vi "VisualizeAppRingdown.vi"() -> ()   [LabVIEW 2017, in "Visualization.lvlib" / "VisualizeAppRingdown.lvclass"]
uses:
  VisualizeAppRingdown.lvclass
  Modules/AppPlugins/RingdownPlugin/PublicAPI/TypeDef/RingdownOutput.ctl
  C:/dev/Work/PARTF/Visualization/VisualizeApp_class/VisualizeAppBase_class.lvclass
  Modules/AppModule/PublicAPI/Arguments/Broadcasts/clStatUpdate.ctl
  VisializeBase_class/Requests/clUserEventType.ctl
  Modules/EventPlugins/EventPluginBaseClass/TypeDefs/clEvtReportArray.ctl
  Modules/EventPlugins/EventPluginBaseClass/TypeDefs/clEvtReport.ctl
  VisualizeAppBase_class.lvclass/VisualizeAppBase_class.ctl
  VisualizeAppRingdown.lvclass/VisualizeAppRingdown.ctl
  <vilib>/event_ctls.llb/usereventprio.ctl
  VisualizeAppBase/Accessors/Write clEvtReportArray.vi
  Accessors/Write EvtParams.vi
  Accessors/Read EvtParams.vi
  VisualizeAppBase/Accessors/Read clEvtReportArray.vi
  Accessors/Write AppOutput.vi
  Accessors/Read AppOutput.vi
  <vilib>/Utility/error.llb/Error Cluster From Error Code.vi
  <vilib>/express/express shared/transition.llb/Dynamic To Waveform Array.vi
  <vilib>/express/express signal manip/GetorSetDDTAttributes/Set DDT Attributes/SetT0.vi
  <vilib>/express/express shared/transition.llb/Waveform Array To Dynamic.vi
  <vilib>/ErrorRing/Error Ring.xnode
  <vilib>/express/express signal manip/GetorSetDDTAttributes/Set DDT Attributes/Set DDT Properties.xnode
  <userlib>/NIST/NISTErrorLib/NISTErrorLib.lvlib
  VisializeBase_class/VisualizeBase_class.lvclass
  Modules/AppModule/AppModule.lvlib
  Modules/EventPlugins/EventPluginBaseClass/EventPluginBaseClass.lvclass
  Modules/AppPlugins/RingdownPlugin/RingdownPlugin.lvclass
  Modules/PmuImpairModule/PmuImpairModule.lvlib
  Modules/EventModule/EventModule.lvlib
panel:
  out "ActivePlot":u32=1
  out "Timeoffset":dbl=1e+32
  in  "restart VI":bool
  out "Error Array":errorcluster[][](array[cluster])
  out "Active Power Signal":dynamicdata(graph)
  out "Error signal":waveform(dbl)[](graph)
  out "S Plane":cluster{"Damping":dbl[], "Frequency":dbl[]}[](graph)
  in  "Number of Visible Modes":dbl=5.0
  out "Input Data":dbl[][](array[numeric])
  out "data 2":T1
  in  "QueName":string="VisAppQue"
  in  "btnStop":bool
  out "Status Broadcasts":string
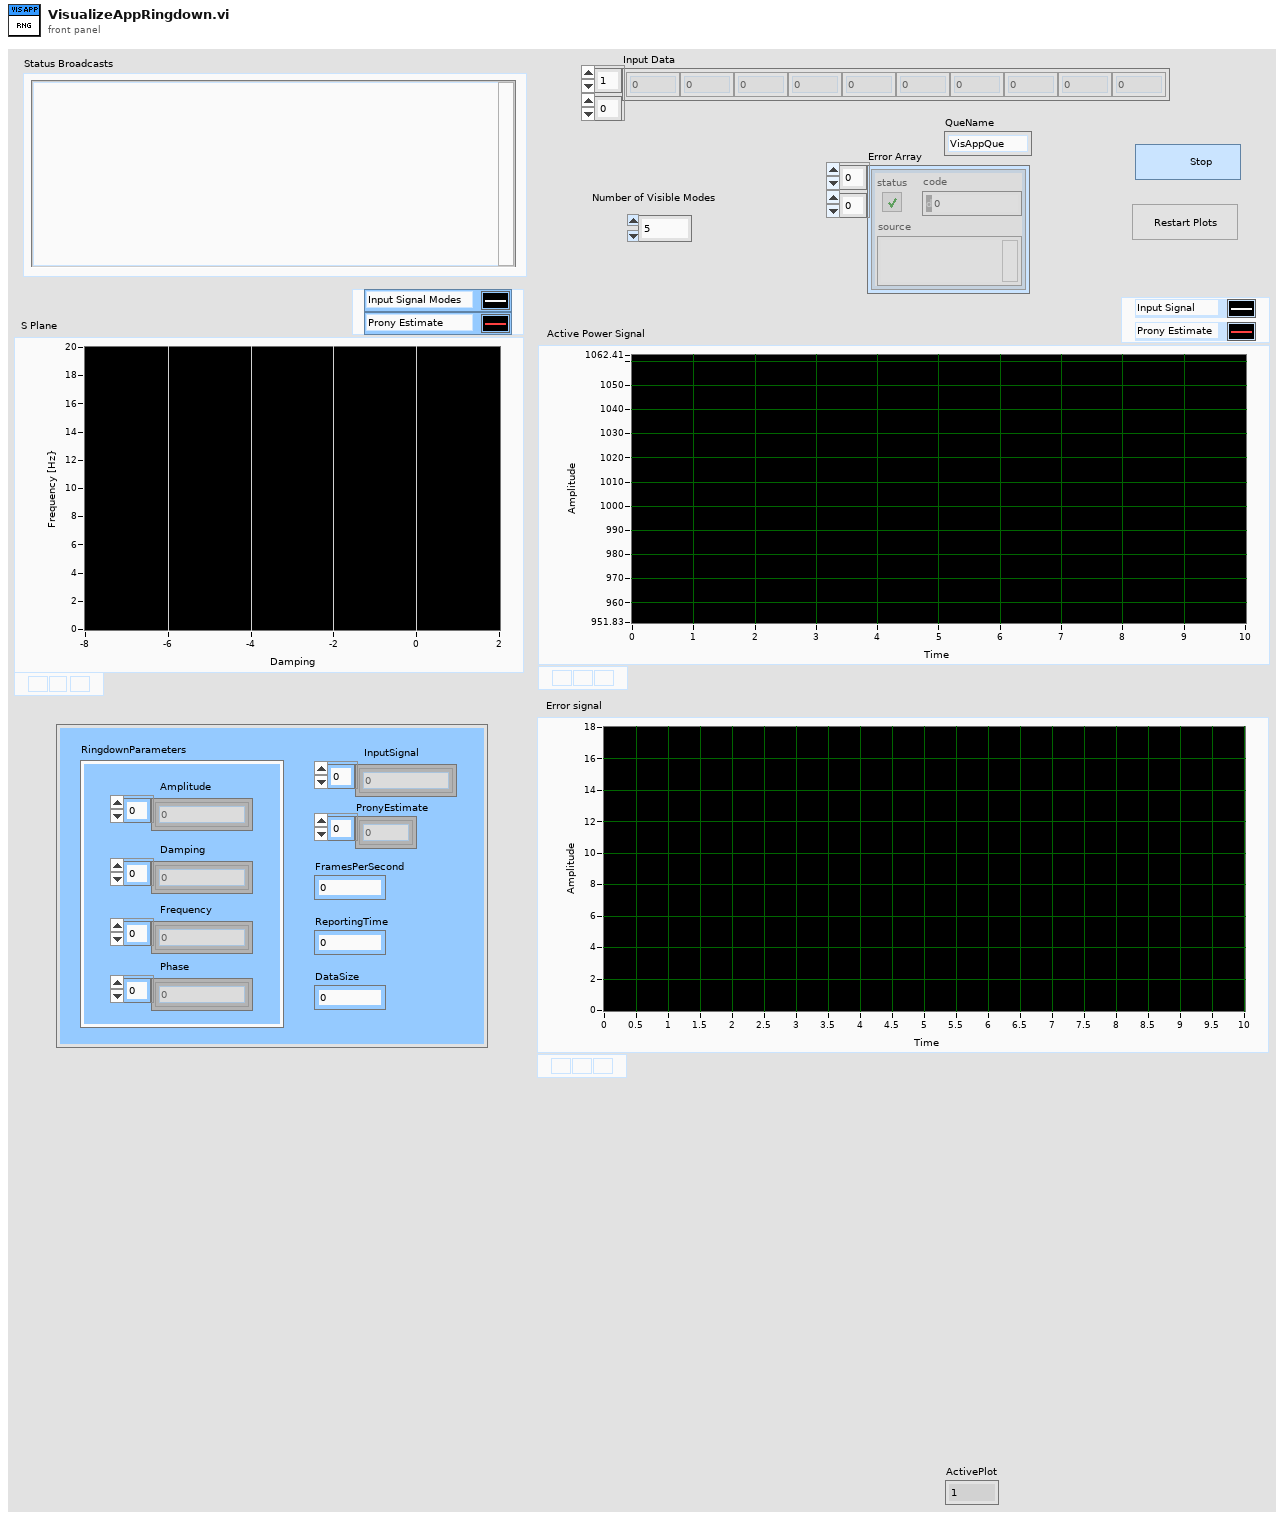
[diagram p1: front panel]
types:
  T1 = typedef "AppPlugins.lvlib/RingdownPlugin.lvclass/RingdownOutput.ctl" = cluster{"FramesPerSecond":dbl, "PronyEstimate":dbl[], "RingdownParameters":cluster{"Amplitude":dbl[], "Damping":dbl[], "Frequency":dbl[], "Phase":dbl[]}, "ReportingTime":dbl, "DataSize":u32, "InputSignal":dbl[]}
  T2 = typedef "EventPlugins.lvlib/EventPluginBaseClass.lvclass/clEvtReportArray.ctl" = T3[]
  T3 = typedef "EventPlugins.lvlib/EventPluginBaseClass.lvclass/clEvtReport.ctl" = cluster{"Timestamp":dbl, "Synx":cdb[], "Freq":dbl, "ROCOF":dbl, "ID":i16}
  T4 = typedef "Visualization.lvlib/VisualizeBase_class.lvclass/clUserEventType.ctl" = cluster{"BusIndex":i8, "Data":variant}
  T5 = typedef "usereventprio.ctl" = enum32{"high priority", "normal priority"}
  T6 = typedef "AppModule.lvlib/clStatUpdate.ctl" = cluster{"Status":string}
  T7 = typedef "Visualization.lvlib/VisualizeBase_class.lvclass/clRequestEvents.ctl" = cluster{"StopRequest":refnum<user-event>}
  T8 = typedef "AppModule.lvlib/clBroadcastEvents.ctl" = cluster{"DidInit":refnum<user-event>, "StatusUpdate":refnum<user-event>, "ErrorReport":refnum<user-event>, "DidStop":refnum<user-event>, "PathToINI":refnum<user-event>, "InputData":refnum<user-event>, "OutputData":refnum<user-event>, "BcAppInfo":refnum<user-event>, "ConfigData":refnum<user-event>}
  T9 = typedef "PmuImpairModule.lvlib/clBroadcastEvents.ctl" = cluster{"DidInit":refnum<user-event>, "StatusUpdate":refnum<user-event>, "ErrorReport":refnum<user-event>, "DidStop":refnum<user-event>, "ImpairConfig":refnum<user-event>, "ImpairParams":refnum<user-event>, "ImpairReports":refnum<user-event>, "PathToPlugin":refnum<user-event>, "BusNumber":refnum<user-event>}
  T10 = typedef "EventModule.lvlib/clBroadcastEvents.ctl" = cluster{"DidInit":refnum<user-event>, "StatusUpdate":refnum<user-event>, "ErrorReport":refnum<user-event>, "DidStop":refnum<user-event>, "ReadEvtConfig":refnum<user-event>, "ReadTimeArray":refnum<user-event>, "ReadEvtParams":refnum<user-event>, "GetEvtReportArray":refnum<user-event>, "ReadPathToPlugin":refnum<user-event>, "GetEvtSignal":refnum<user-event>, "ReadBusNumber":refnum<user-event>}
  T11 = cluster{"Amplitude":dbl[], "Damping":dbl[], "Frequency":dbl[], "Phase":dbl[]}
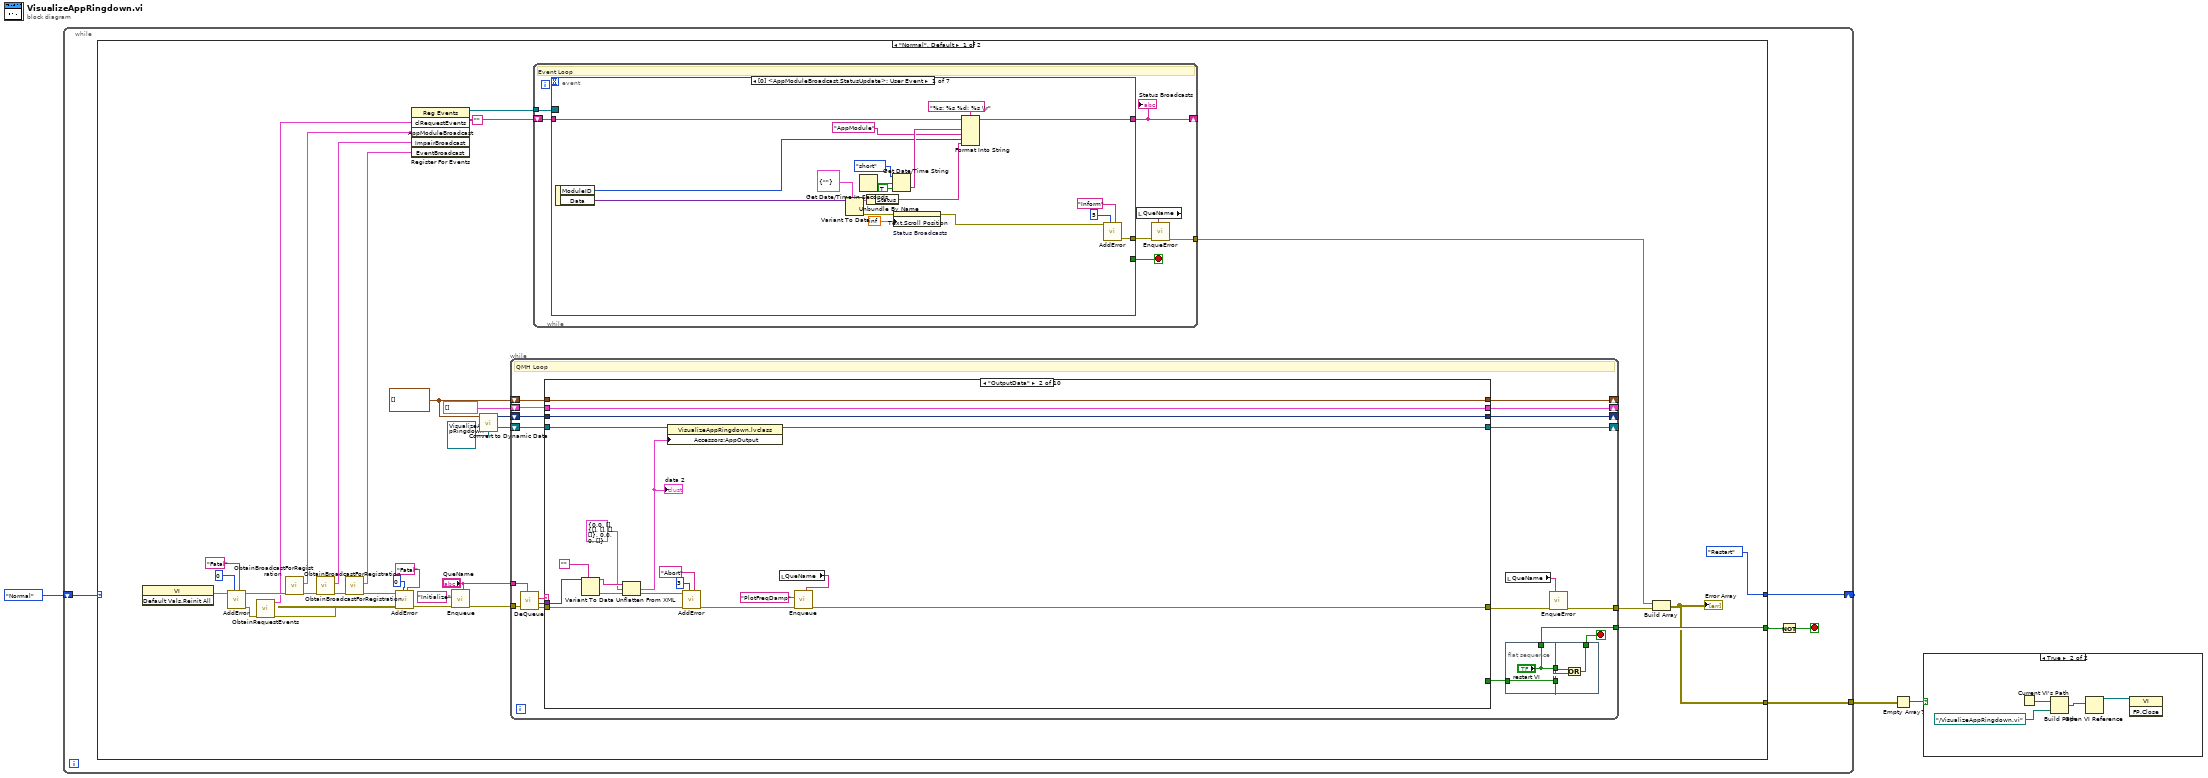
[diagram p0: block diagram]
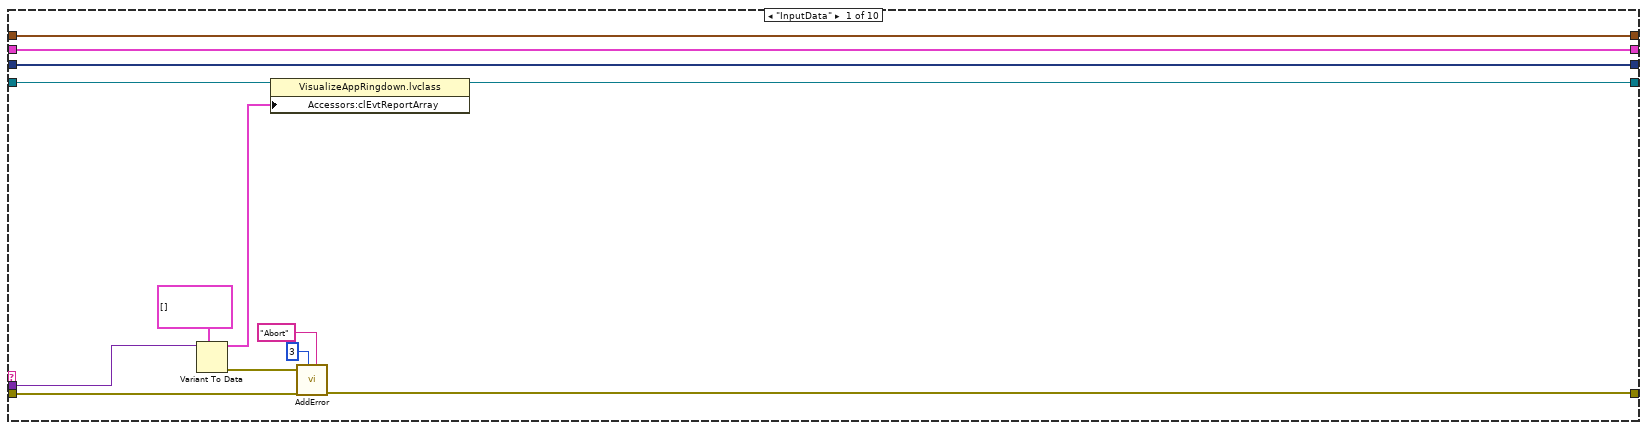
[diagram p3: hidden frame]
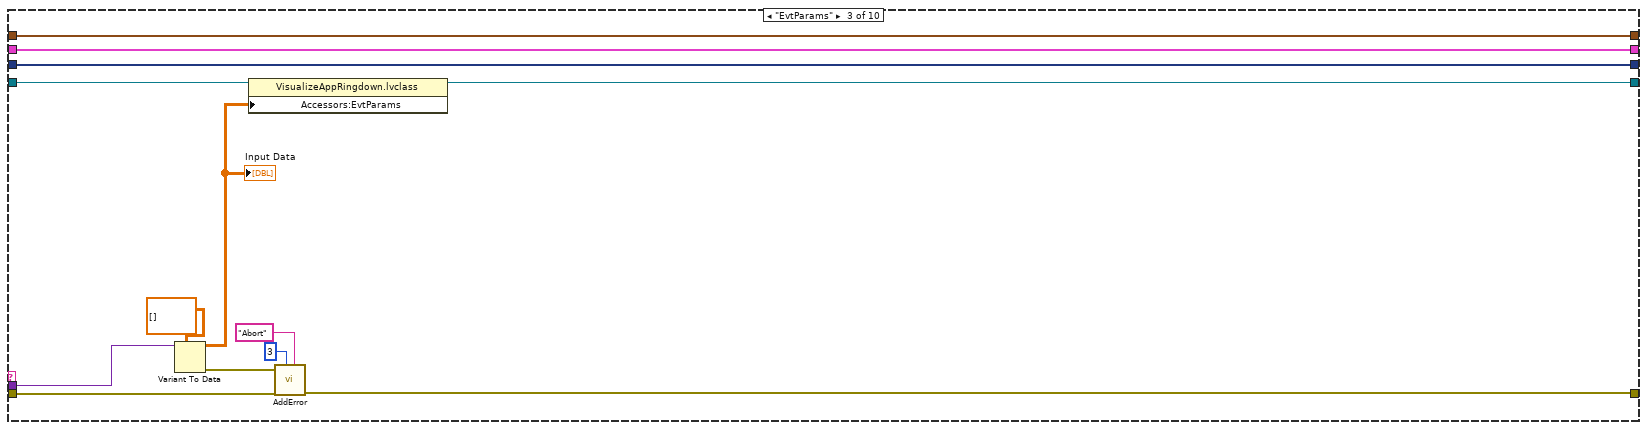
[diagram p4: hidden frame]
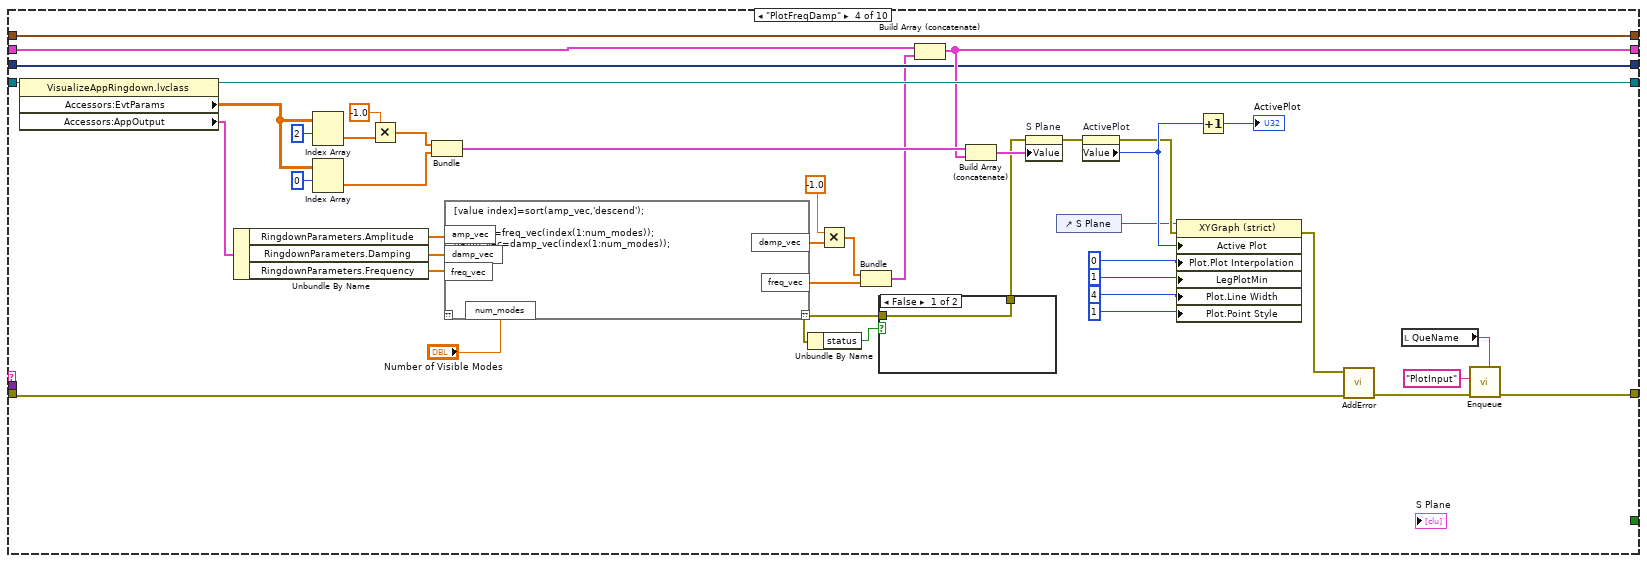
[diagram p5: hidden frame]
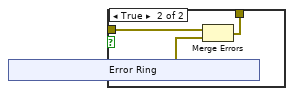
[diagram p6: hidden frame]
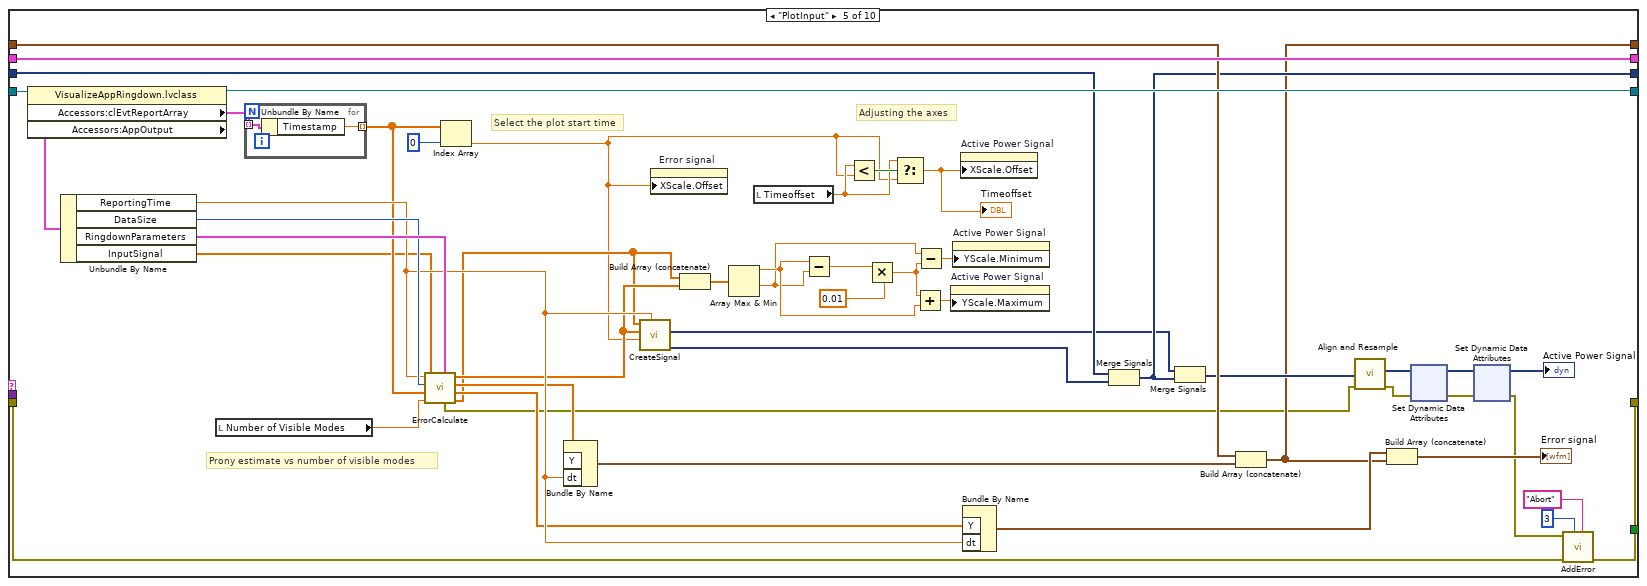
[diagram p7: hidden frame]
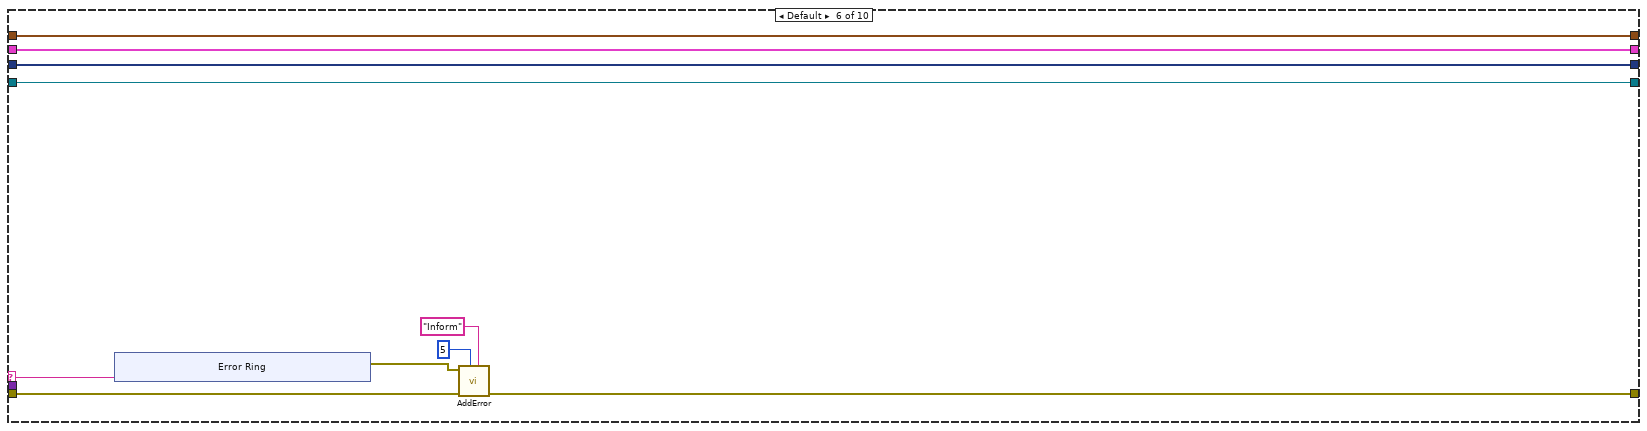
[diagram p8: hidden frame]
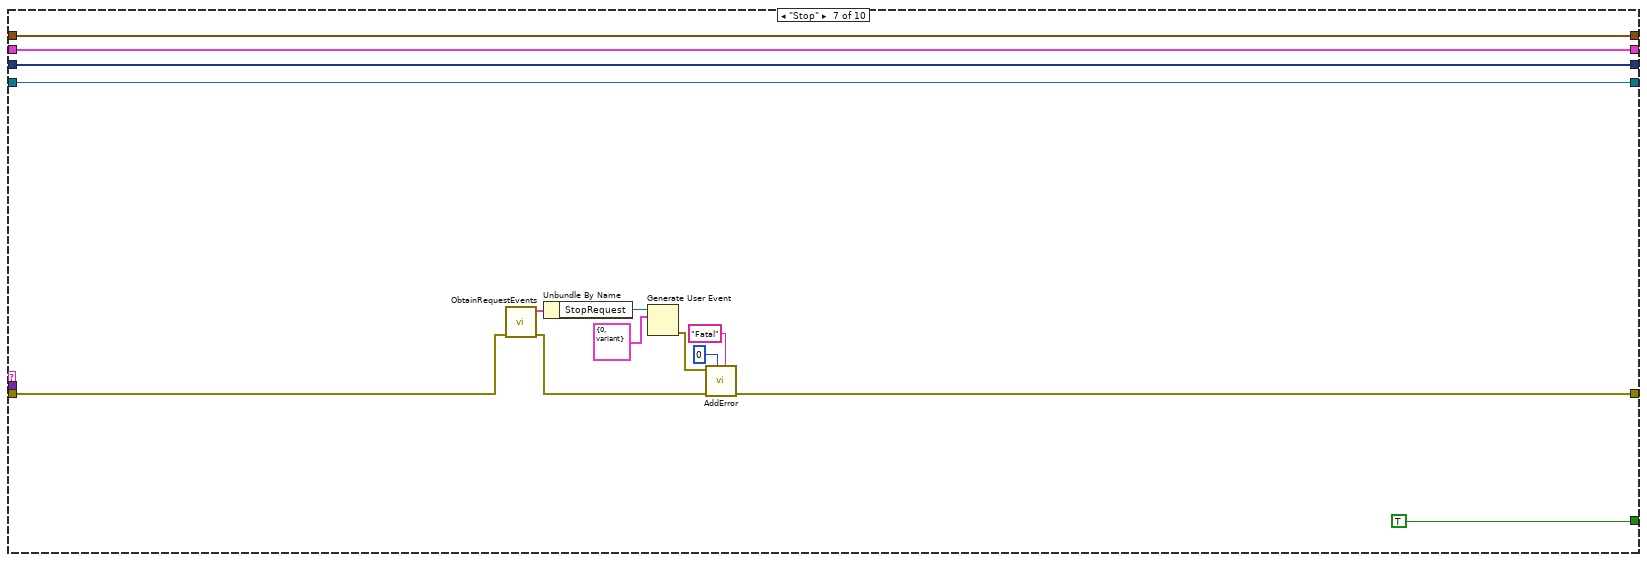
[diagram p9: hidden frame]
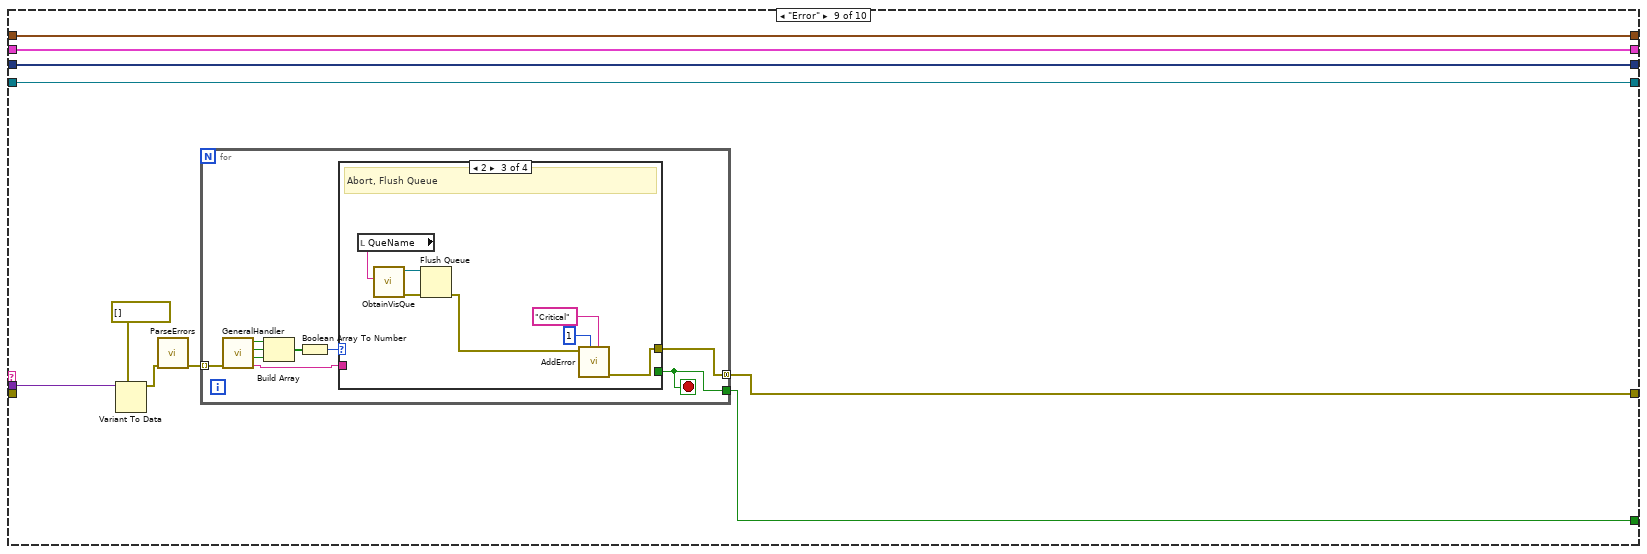
[diagram p11: hidden frame]
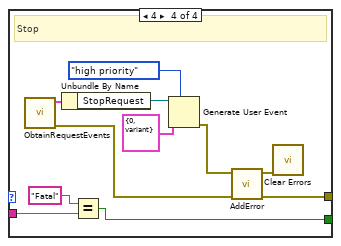
[diagram p14: hidden frame]
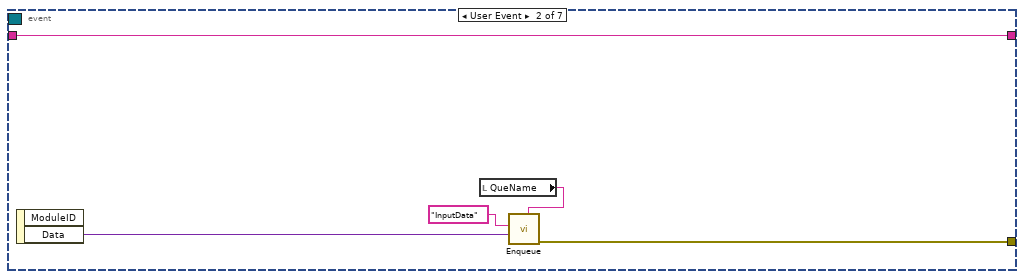
[diagram p16: hidden frame]
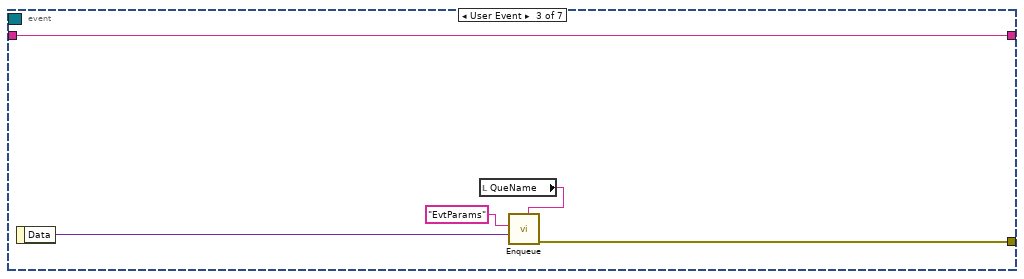
[diagram p17: hidden frame]
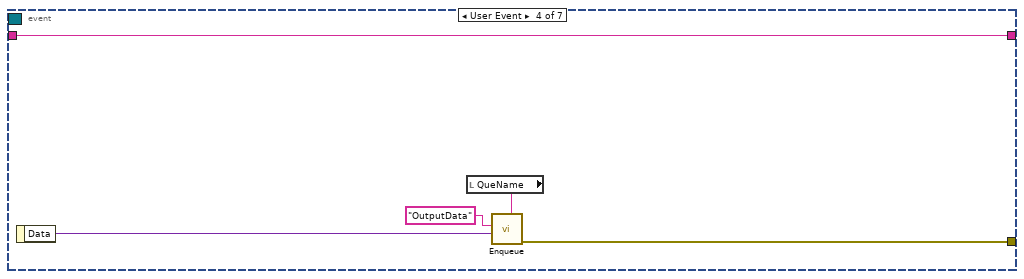
[diagram p18: hidden frame]
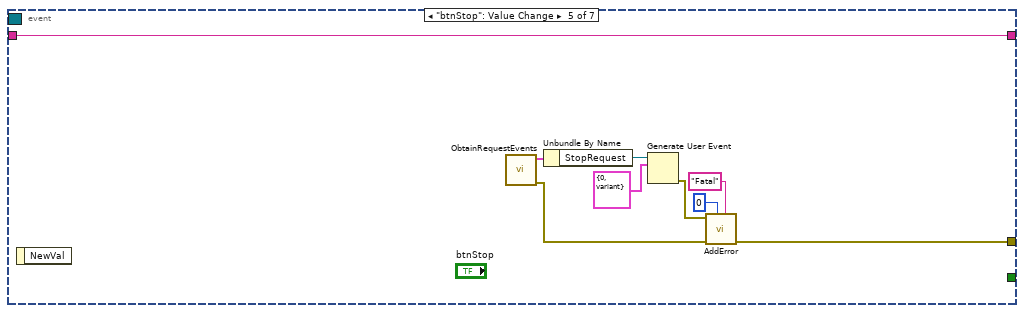
[diagram p19: hidden frame]
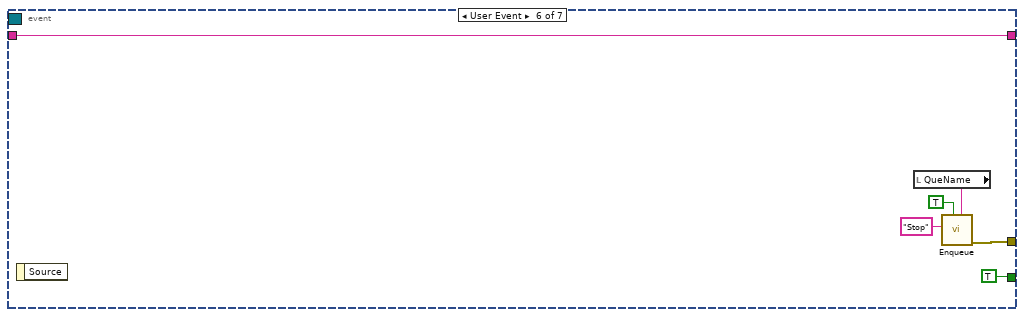
[diagram p20: hidden frame]
diagram:
  n1 = while {
    shift-right: [w5] -> _
    shift-left: enum16{"Normal", "Restart"}."Normal" -> [w6]
    tunnel: [w4] -> w1
    stop <- w7 stop-if-true
    n2 = case shown="\"Normal\", Default" w6 {
      tunnel: [w13 TRUE] -> w8
      tunnel: [enum16{"Normal", "Restart"}."Restart" enum16{"Normal", "Restart"}."Normal"] -> w5
      tunnel: [w9 errorcluster[][] []] -> w4
      frame "Normal", Default {
        w11 = waveform(dbl)[] []
        n3 = invoke class="VI" method="Default Vals.Reinit All"() -> (error out=w21:errorcluster)  [unwired: 3 in, 2 out]
        n4 = call <userlib>:"AddError.vi"("Severity"="Fatal", "Priority"=u8 0, "error in (no error)"=w21) -> ("ErrorArray"=w36:errorcluster[], "error out"=w35:errorcluster)  [unwired: 7 in]
        n5 = call "ObtainRequestEvents.vi"("Error"=w36) -> ("Error"=w32:errorcluster[], "clRequestEvents"=w34:T7)  [unwired: 9 in]
        n6 = call "ObtainBroadcastForRegistration.vi"("error in (no error)"=w35) -> ("error out"=w20:errorcluster, "AppModuleBroadcast"=w33:T8)  [unwired: 9 in]
        n7 = call "ObtainBroadcastForRegistration.vi"("error in (no error)"=w20) -> ("error out"=w19:errorcluster, "ImpairBroadcast"=w18:T9)  [unwired: 9 in]
        n8 = call "ObtainBroadcastForRegistration.vi"("error in (no error)"=w19) -> ("error out"=w16:errorcluster, "EventBroadcast"=w15:T10)  [unwired: 9 in]
        n9 = call <userlib>:"AddError.vi"("Severity"="Fatal", "Priority"=u8 0, "ErrorArray"=w32, "error in (no error)"=w16) -> ("ErrorArray"=w30:errorcluster[])  [unwired: 6 in, 1 out]
        n10 = register-events(w34, w33, w18, w15) -> (reference out=w25:refnum<event-registration>)  [unwired: 2 in, 1 out]
        n11 = call "Enqueue.vi"("QueName"="QueName", "Error"=w30, "Message"="Initialize") -> ("Error"=w27:errorcluster[])  [unwired: 8 in]
        n12 = call "Convert to Dynamic Data"("Array of Waveforms"=w11) -> ("Dynamic Data Type"=w10:dynamicdata)  [unwired: 3 in]
        n13 = while {
          tunnel: w27 -> [w59]
          tunnel: "QueName" -> [w58]
          tunnel: [w52] -> w24
          shift-right: [w50] -> _
          shift-left: refnum<class "VisualizeAppRingdown.lvclass"> refnum ("Visualization.lvlib:VisualizeAppRingdown.lvclass") -> [w51]
          shift-right: [w49] -> _
          shift-left: cluster{"Damping":dbl[], "Frequency":dbl[]}[] [] -> [w48]
          shift-right: [w46] -> _
          shift-left: w10 -> [w47]
          shift-right: [w44] -> _
          shift-left: w11 -> [w45]
          tunnel: [w43] -> w13
          stop <- w39 stop-if-true
          # "QMH Loop"
          n14 = call "DeQueue.vi"("QueName"=w58, "Error"=w59) -> ("Error"=w55:errorcluster[], "Data"=w56:variant, "Message"=w57:string)  [unwired: 7 in]
          n15 = case shown="\"OutputData\"" w57 {
            selector: w57 -> [_ _ _ _ _ w250 _ _ _ _]
            tunnel: w56 -> [w75 w94 w107 _ _ _ _ _ w283 _]
            tunnel: w55 -> [w71 w93 w104 w122 w174 w249 w263 w276 _ w314]
            tunnel: [w70 w89 w103 w119 w173 w245 w264 w276 w285 w314] -> w54
            tunnel: [_ _ _ _ _ _ TRUE _ w286 _] -> w41
            tunnel: w51 -> [w77 w96 w109 w152 w210 w244 w261 w275 w280 w315]
            tunnel: [w76 w95 w108 w151 w209 w244 w261 w275 w280 w315] -> w50
            tunnel: [w67 w86 w99 w143 w208 w243 w260 w274 w279 w317] -> w49
            tunnel: w48 -> [w67 w86 w99 w144 w208 w243 w260 w274 w279 w317]
            tunnel: w47 -> [w66 w85 w98 w142 w201 w242 w259 w273 w278 w316]
            tunnel: [w66 w85 w98 w142 w200 w242 w259 w273 w278 w316] -> w46
            tunnel: w45 -> [w65 w84 w97 w140 w205 w241 w258 w272 w277 w318]
            tunnel: [w65 w84 w97 w140 w198 w241 w258 w272 w277 w318] -> w44
            frame "InputData" {
              n16 = Variant To Data(type=T2 [] ("clEvtReportArray"), Variant=w75) -> (data=w73:T2, error out=w72:errorcluster)  [unwired: 1 in]
              n17 = property class="VisualizeAppRingdown.lvclass"(reference=w77, "Accessors:clEvtReportArray"=w73) -> (reference out=w76:refnum<class "VisualizeAppRingdown.lvclass">)  [unwired: 1 in, 1 out]
              n18 = call <userlib>:"AddError.vi"("Severity"="Abort", "Priority"=u8 3, "ErrorArray"=w71, "error in (no error)"=w72) -> ("ErrorArray"=w70:errorcluster[])  [unwired: 6 in, 1 out]
            }
            frame "OutputData" {
              n19 = Variant To Data(type="", Variant=w94) -> (data=w83:string, error out=w80:errorcluster)  [unwired: 1 in]
              n20 = Unflatten From XML(xml string=w83, type=T1 {"FramesPerSecond"=0.0, "PronyEstimate"=[], "RingdownParameters"={"Amplitude"=[], "Damping"=[], "Frequency"=[], "Phase"=[]}, "ReportingTime"=0.0, "DataSize"=0, "InputSignal"=[]} ("RingdownOutput"), error in (no error)=w80) -> (value=w78:T1, error out=w79:errorcluster)
              "data 2" <- w78
              n21 = property class="VisualizeAppRingdown.lvclass"(reference=w96, "Accessors:AppOutput"=w78) -> (reference out=w95:refnum<class "VisualizeAppRingdown.lvclass">)  [unwired: 1 in, 1 out]
              n22 = call <userlib>:"AddError.vi"("Severity"="Abort", "Priority"=u8 3, "ErrorArray"=w93, "error in (no error)"=w79) -> ("ErrorArray"=w90:errorcluster[])  [unwired: 6 in, 1 out]
              n23 = local read "QueName"() -> (w87:string)
              n24 = call "Enqueue.vi"("QueName"=w87, "Error"=w90, "Message"="PlotFreqDamp") -> ("Error"=w89:errorcluster[])  [unwired: 8 in]
            }
            frame "EvtParams" {
              n25 = Variant To Data(type=dbl[][] [], Variant=w107) -> (data=w106:dbl[][], error out=w105:errorcluster)  [unwired: 1 in]
              "Input Data" <- w106
              n26 = property class="VisualizeAppRingdown.lvclass"(reference=w109, "Accessors:EvtParams"=w106) -> (reference out=w108:refnum<class "VisualizeAppRingdown.lvclass">)  [unwired: 1 in, 1 out]
              n27 = call <userlib>:"AddError.vi"("Severity"="Abort", "Priority"=u8 3, "ErrorArray"=w104, "error in (no error)"=w105) -> ("ErrorArray"=w103:errorcluster[])  [unwired: 6 in, 1 out]
            }
            frame "PlotFreqDamp" {
              n28 = property class="VisualizeAppRingdown.lvclass"(reference=w152) -> (reference out=w151:refnum<class "VisualizeAppRingdown.lvclass">, "Accessors:EvtParams"=w148:dbl[][], "Accessors:AppOutput"=w150:T1)  [unwired: 1 in, 1 out]
              n29 = Unbundle By Name(w150) -> ("RingdownParameters.Amplitude"=w132:dbl[], "RingdownParameters.Damping"=w131:dbl[], "RingdownParameters.Frequency"=w130:dbl[])
              n30 = Index Array(array=w148, index (row)=2) -> (element=w139:dbl[])  [unwired: 1 in]
              n31 = Index Array(array=w148, index (row)=0) -> (element=w146:dbl[])  [unwired: 1 in]
              n32 = Multiply(x=-1.0, y=w139) -> (x*y=w138:dbl[])
              n33 = Bundle(w138, "Accessors:EvtParams"=w146) -> (w145:cluster{dbl[], "Accessors:EvtParams":dbl[]})  [unwired: 1 in]
              n34 = script code="[value index]=sort(amp_vec,'descend');\n\nfreq_vec=freq_vec(index(1:num_modes));\ndamp_vec=damp_vec(index(1:num_modes));"("amp_vec"=w132, "damp_vec"=w131, "freq_vec"=w130, "num_modes"="Number of Visible Modes") -> ("??"=w111:errorcluster, "damp_vec"=w134:dbl[], "freq_vec"=w133:dbl[])  [unwired: 1 in]
              n35 = Unbundle By Name(w111) -> ("status"=w110:bool)
              n36 = Multiply(x=-1.0, y=w134) -> (x*y=w135:dbl[])
              n37 = Bundle(w135, w133) -> (w141:cluster{dbl[], dbl[]})  [unwired: 1 in]
              n38 = case shown="False" w110 {
                tunnel: [w153 w156] -> w112
                tunnel: w111 -> [w153 w154]
                frame False {
                }
                frame True {
                  n39 = xnode "Error Ring"() -> ("error out"=w155:errorcluster)
                  n40 = Merge Errors(w154, w155) -> (w156:errorcluster)
                }
              }
              n41 = Build Array (concatenate)(w144, w141) -> (w143:cluster{"Damping":dbl[], "Frequency":dbl[]}[])
              n42 = Build Array (concatenate)(w145, w143) -> (w127:cluster{"Damping":dbl[], "Frequency":dbl[]}[])
              n43 = property on="S Plane" class="XYGraph (strict)"(error in=w112, "Value"=w127) -> (error out=w126:errorcluster)  [unwired: 1 in, 1 out]
              n44 = control-ref of="S Plane"() -> (w113:refnum<vi>)
              n45 = property on="ActivePlot" class="DigNum (strict)"(error in=w126) -> (error out=w124:errorcluster, "Value"=w125:u32)  [unwired: 1 in, 1 out]
              n46 = property on="Property Node" class="XYGraph (strict)"(reference=w113, error in=w124, "Active Plot"=w125, "Plot.Plot Interpolation"=u8 0, "LegPlotMin"=u32 1 ("Legend:Plot Minimum"), "Plot.Line Width"=u8 4, "Plot.Point Style"=u8 1) -> (error out=w123:errorcluster)  [unwired: 1 out]
              n47 = Increment(x=w125) -> (x+1=→"ActivePlot":u32)
              n48 = call <userlib>:"AddError.vi"("ErrorArray"=w122, "error in (no error)"=w123) -> ("ErrorArray"=w120:errorcluster[])  [unwired: 8 in, 1 out]
              n49 = local read "QueName"() -> (w118:string)
              n50 = call "Enqueue.vi"("QueName"=w118, "Error"=w120, "Message"="PlotInput") -> ("Error"=w119:errorcluster[])  [unwired: 8 in]
            }
            frame "PlotInput" {
              # "Adjusting the axes"
              # "Select the plot start time"
              # "Prony estimate vs number of visible modes"
              n51 = property class="VisualizeAppRingdown.lvclass"(reference=w210) -> (reference out=w209:refnum<class "VisualizeAppRingdown.lvclass">, "Accessors:clEvtReportArray"=w193:T2, "Accessors:AppOutput"=w207:T1)  [unwired: 1 in, 1 out]
              n52 = Unbundle By Name(w207) -> ("ReportingTime"=w178:dbl, "DataSize"=w179:u32, "RingdownParameters"=w180:T11, "InputSignal"=w164:dbl[])
              n53 = local read "Number of Visible Modes"() -> (w166:dbl)
              n54 = for {
                tunnel: w193 -> [w240] mode=indexing
                tunnel: [w239] -> w167 mode=indexing
                n55 = Unbundle By Name(w240) -> ("Timestamp"=w239:dbl)
              }
              n56 = call "ErrorCalculate.vi"("RingdownParameters"=w180, "input_data"=w164, "num_modes"=w166, "time"=w167, "nnfit"=w179, "dft"=w178) -> ("input_data"=w163:dbl[], "null_input"=w177:dbl[], "error_sig"=w175:dbl[], "prony_estimate"=w176:dbl[], "error out"=w165:errorcluster)  [unwired: 1 in]
              n57 = Index Array(array=w167, index=0) -> (element=w162:dbl)
              n58 = Bundle By Name("Y"=w175, "dt"=w178) -> (w206:waveform(dbl))  [unwired: 1 in]
              n59 = call "CreateSignal.vi"("dt"=w178, "t0_1"=w162, "PronyEstimate"=w176, "InputSignal"=w163) -> ("DynamicPronyEstimate"=w181:dynamicdata, "DynamicInputSignal"=w182:dynamicdata)  [unwired: 6 in]
              n60 = property on="Error signal" class="WFGraph (strict)"("XScale.Offset"=w162) -> ()  [unwired: 2 in, 2 out]
              n61 = Build Array (concatenate)(w163, w176) -> (w186:dbl[])
              n62 = Array Max & Min(array=w186) -> (max value=w190:dbl, min value=w189:dbl)  [unwired: 2 out]
              n63 = local read "Timeoffset"() -> (w196:dbl)
              n64 = Subtract(x=w190, y=w189) -> (x-y=w188:dbl)
              n65 = Less?(x=w196, y=w162) -> (x < y?=w197:bool)
              n66 = Multiply(x=w188, y=0.01) -> (x*y=w187:dbl)
              n67 = Select(t=w196, s=w197, f=w162) -> (s? t:f=w194:dbl)
              "Timeoffset" <- w194
              n68 = Add(x=w187, y=w190) -> (x+y=w192:dbl)
              n69 = Subtract(x=w189, y=w187) -> (x-y=w195:dbl)
              n70 = property on="Active Power Signal" class="WFGraph (strict)"("YScale.Maximum"=w192) -> ()  [unwired: 2 in, 2 out]
              n71 = property on="Active Power Signal" class="WFGraph (strict)"("YScale.Minimum"=w195) -> ()  [unwired: 2 in, 2 out]
              n72 = property on="Active Power Signal" class="WFGraph (strict)"("XScale.Offset"=w194) -> ()  [unwired: 2 in, 2 out]
              n73 = Bundle By Name("Y"=w177, "dt"=w178) -> (w203:waveform(dbl))  [unwired: 1 in]
              n74 = Merge Signals(w201, w181) -> (w200:dynamicdata)
              n75 = Merge Signals(w182, w200) -> (w199:dynamicdata)
              n76 = Build Array (concatenate)(w205, w206) -> (w198:waveform(dbl)[])
              n77 = call "Align and Resample"("error in (no error)"=w165, "Signals"=w199) -> ("error out"=w172:errorcluster, "Resampled Signals"=w185:dynamicdata)  [unwired: 7 in, 1 out]
              n78 = Build Array (concatenate)(w203, w198) -> (→"Error signal":waveform(dbl)[])
              n79 = xnode "Set Dynamic Data Attributes"("Signals In"=w185, "error in"=w172) -> ("Signals Out"=w184:dynamicdata, "error out"=w171:errorcluster)  [unwired: 2 in]
              n80 = xnode ("Set Dynamic Data Attributes")("Signals In"=w184, "error in"=w171) -> ("Signals Out"=→"Active Power Signal":dynamicdata, "error out"=w170:errorcluster)  [unwired: 2 in]
              n81 = call <userlib>:"AddError.vi"("Severity"="Abort", "Priority"=u8 3, "ErrorArray"=w174, "error in (no error)"=w170) -> ("ErrorArray"=w173:errorcluster[])  [unwired: 6 in, 1 out]
            }
            frame Default {
              n82 = xnode "Error Ring"("parameter 0"=w250) -> ("error out"=w248:errorcluster)
              n83 = call <userlib>:"AddError.vi"("Severity"="Inform", "Priority"=u8 5, "ErrorArray"=w249, "error in (no error)"=w248) -> ("ErrorArray"=w245:errorcluster[])  [unwired: 6 in, 1 out]
            }
            frame "Stop" {
              n84 = call "ObtainRequestEvents.vi"("Error"=w263) -> ("Error"=w262:errorcluster[], "clRequestEvents"=w265:T7)  [unwired: 9 in]
              n85 = Unbundle By Name(w265) -> ("StopRequest"=w266:refnum<user-event>)
              n86 = Generate User Event(user event=w266, event data cluster=T4 {"BusIndex"=0, "Data"=variant} ("clEventType")) -> (error out=w268:errorcluster)  [unwired: 2 in, 1 out]
              n87 = call <userlib>:"AddError.vi"("Severity"="Fatal", "Priority"=u8 0, "ErrorArray"=w262, "error in (no error)"=w268) -> ("ErrorArray"=w264:errorcluster[])  [unwired: 6 in, 1 out]
            }
            frame "Initialize" {
            }
            frame "Error" {
              n88 = Variant To Data(type=errorcluster[] [], Variant=w283) -> (data=w281:errorcluster[])  [unwired: 1 in, 1 out]
              n89 = call <userlib>:"ParseErrors.vi"("ErrorArray"=w281) -> ("ErrorArray"=w284:errorcluster[])  [unwired: 8 in, 2 out]
              n90 = for {
                tunnel: w284 -> [w295] mode=indexing
                tunnel: [w289] -> w285 mode=concatenating
                tunnel: [w287] -> w286
                stop <- w287 stop-if-true
                n91 = call <userlib>:"GeneralHandler.vi"("error in (no error)"=w295) -> ("Severity"=w288:string, "Stop"=w292:bool, "Abort"=w293:bool, "Continue"=w294:bool)  [unwired: 7 in]
                n92 = Build Array(w294, w293, w292) -> (w291:bool[])
                n93 = Boolean Array To Number(Boolean array=w291) -> (number=w290:u32)
                n94 = case shown="2" w290 {
                  tunnel: [_ _ w300 w311] -> w289
                  tunnel: w288 -> [_ _ _ w305]
                  tunnel: [_ _ _ w303] -> w287
                  frame 0, Default {
                    # "No Dialog"
                  }
                  frame 1 {
                    # "Continue"
                  }
                  frame 2 {
                    # "Abort, Flush Queue"
                    n95 = local read "QueName"() -> (w296:string)
                    n96 = call "ObtainVisQue.vi"("QueName"=w296) -> ("error out"=w302:errorcluster, "queue out"=w301:refnum<queue>)  [unwired: 9 in]
                    n97 = Flush Queue(queue=w301, error in (no error)=w302) -> (error out=w299:errorcluster)  [unwired: 2 out]
                    n98 = call <userlib>:"AddError.vi"("Severity"="Critical" ("String"), "Priority"=u8 1, "error in (no error)"=w299) -> ("ErrorArray"=w300:errorcluster[])  [unwired: 7 in, 1 out]
                  }
                  frame 4 {
                    # "Stop"
                    n99 = call "ObtainRequestEvents.vi"() -> ("Error"=w309:errorcluster[], "clRequestEvents"=w313:T7)  [unwired: 10 in]
                    n100 = Unbundle By Name(w313) -> ("StopRequest"=w312:refnum<user-event>)
                    n101 = Equal?(x="Fatal", y=w305) -> (x = y?=w303:bool)
                    n102 = Generate User Event(priority (normal)=usereventprio."high priority", user event=w312, event data cluster=T4 {"BusIndex"=0, "Data"=variant} ("event data")) -> (error out=w310:errorcluster)  [unwired: 1 in, 1 out]
                    n103 = call <userlib>:"AddError.vi"("ErrorArray"=w309, "error in (no error)"=w310) -> ("ErrorArray"=w311:errorcluster[], "error out"=w306:errorcluster)  [unwired: 8 in]
                    n104 = call <vilib>:"Clear Errors.vi"("error in (no error)"=w306) -> ()  [unwired: 5 in, 2 out]
                  }
                }
              }
            }
            frame "Restart" {
            }
          }
          n105 = flat-sequence {
            tunnel: ["restart VI"] -> w43
            tunnel: ["restart VI"] -> w42
            tunnel: w41 -> [w60]
            tunnel: [w60] -> w40
            tunnel: w42 -> [w64]
            tunnel: w40 -> [w63]
            tunnel: [w62] -> w39
            frame #0 {
            }
            frame #1 {
              n106 = Or(x=w63, y=w64) -> (x .or. y?=w62:bool)
            }
          }
          n107 = local read "QueName"() -> (w53:string)
          n108 = call "EnqueError.vi"("QueName"=w53, "Error"=w54) -> ("Error"=w52:errorcluster[])  [unwired: 9 in]
        }
        n109 = while {
          tunnel: [w324] -> w23
          tunnel: w25 -> [w322]
          shift-right: [w319] -> _
          shift-left: "" -> [w320]
          stop <- w321 stop-if-true
          # "Event Loop"
          n110 = event shown="[0] <AppModuleBroadcast.StatusUpdate>: User Event" {
            selector: w322 -> [_ _ _ _ _ _ _]
            dyn-events: _ -> [_ _ _ _ _ _ _]
            timeout: _ -> [_ _ _ _ _ _ _]
            tunnel: [w333 w348 w353 w358 w363 w371 w375] -> w325
            tunnel: [_ _ _ _ _ TRUE TRUE] -> w321
            tunnel: w320 -> [w344 w346 w351 w355 w360 w369 w380]
            tunnel: [w337 w346 w351 w355 w360 w369 w380] -> w319
            event User Event {
              n111 = event-data() -> ("ModuleID"=w327:i32, "Data"=w343:variant)  [unwired: 1 in]
              n112 = Variant To Data(type=T6 {"Status"=""} ("clStatUpdate"), Variant=w343) -> (data=w341:T6, error out=w334:errorcluster)  [unwired: 1 in]
              n113 = Get Date/Time In Seconds() -> (seconds since 1Jan1904=w338:timestamp)
              n114 = Unbundle By Name(w341) -> ("Status"=w328:string)
              n115 = Get Date/Time String(date format (0)=enum16{"short", "long", "abbreviated"}."short", seconds (now)=w338, want seconds? (F)=TRUE) -> (time string=w335:string)  [unwired: 1 out]
              n116 = property on="Status Broadcasts" class="Str"(error in=w334, "Text.Scroll Position"=inf) -> (error out=w332:errorcluster)  [unwired: 1 in, 1 out]
              n117 = Format Into String(format string="%s: %s %d: %s \\r", initial string=w344, w335, "AppModule", w327, w328) -> (resulting string=w337:string)  [unwired: 1 in, 1 out]
              n118 = call <userlib>:"AddError.vi"("Severity"="Inform", "Priority"=u8 5, "error in (no error)"=w332) -> ("ErrorArray"=w333:errorcluster[])  [unwired: 7 in, 1 out]
            }
            event User Event {
              n119 = event-data() -> ("Data"=w349:variant)  [unwired: 1 in, 1 out]
              n120 = local read "QueName"() -> (w345:string)
              n121 = call "Enqueue.vi"("QueName"=w345, "Data"=w349, "Message"="InputData") -> ("Error"=w348:errorcluster[])  [unwired: 8 in]
            }
            event User Event {
              n122 = event-data() -> ("Data"=w354:variant)  [unwired: 1 in]
              n123 = local read "QueName"() -> (w350:string)
              n124 = call "Enqueue.vi"("QueName"=w350, "Data"=w354, "Message"="EvtParams") -> ("Error"=w353:errorcluster[])  [unwired: 8 in]
            }
            event User Event {
              n125 = event-data() -> ("Data"=w359:variant)  [unwired: 1 in]
              n126 = local read "QueName"() -> (w356:string)
              n127 = call "Enqueue.vi"("QueName"=w356, "Data"=w359, "Message"="OutputData") -> ("Error"=w358:errorcluster[])  [unwired: 8 in]
            }
            event "btnStop": Value Change {
              n128 = event-data() -> ()  [unwired: 1 in, 1 out]
              n129 = call "ObtainRequestEvents.vi"() -> ("Error"=w365:errorcluster[], "clRequestEvents"=w368:T7)  [unwired: 10 in]
              n130 = Unbundle By Name(w368) -> ("StopRequest"=w367:refnum<user-event>)
              n131 = Generate User Event(user event=w367, event data cluster=T4 {"BusIndex"=0, "Data"=variant} ("clEventType")) -> (error out=w364:errorcluster)  [unwired: 2 in, 1 out]
              n132 = call <userlib>:"AddError.vi"("Severity"="Fatal", "Priority"=u8 0, "ErrorArray"=w365, "error in (no error)"=w364) -> ("ErrorArray"=w363:errorcluster[])  [unwired: 6 in, 1 out]
            }
            event User Event {
              n133 = event-data() -> ()  [unwired: 1 in, 1 out]
              n134 = local read "QueName"() -> (w373:string)
              n135 = call "Enqueue.vi"("QueName"=w373, "Priority? (F)"=TRUE, "Message"="Stop") -> ("Error"=w371:errorcluster[])  [unwired: 8 in]
            }
            event "restart VI": Value Change {
              n136 = event-data() -> ()  [unwired: 1 in, 5 out]
              n137 = local read "QueName"() -> (w377:string)
              n138 = call "Enqueue.vi"("QueName"=w377, "Priority? (F)"=TRUE, "Message"="Restart") -> ("Error"=w375:errorcluster[])  [unwired: 8 in]
            }
          }
          "Status Broadcasts" <- w319
          n139 = local read "QueName"() -> (w323:string)
          n140 = call "EnqueError.vi"("QueName"=w323, "Error"=w325) -> ("Error"=w324:errorcluster[])  [unwired: 9 in]
        }
        n141 = Build Array(w23, w24) -> (w9:errorcluster[][])
        "Error Array" <- w9
      }
      frame "Restart" {
        # "Calls the VI server reintializing the VI"
        n142 = control-ref of="This VI"() -> (w382:refnum<vi>)
        n143 = invoke class="VI" method="Default Vals.Reinit All"(reference=w382) -> ()  [unwired: 2 in, 3 out]
      }
    }
    n144 = Not(x=w8) -> (.not. x?=w7:bool)
  }
  n145 = Empty Array?(array=w1) -> (empty?=w2:bool)
  n146 = case shown="True" w2 {
    frame False {
    }
    frame True {
      n147 = Current VI's Path() -> (path=w387:path)
      n148 = Build Path(base path=w387, name or relative path=path "../VisualizeAppRingdown.vi") -> (appended path=w385:path)
      n149 = Open VI Reference(vi path=w385) -> (vi reference=w388:refnum<vi>)  [unwired: 5 in, 1 out]
      n150 = invoke class="VI" method="FP.Close"(reference=w388) -> ()  [unwired: 2 in, 3 out]
    }
  }
